vi "poly_lock_fp_updates_unlock_caller.vi"(8 "error in":errorcluster) -> (0 "error out":errorcluster)   [LabVIEW 2015]
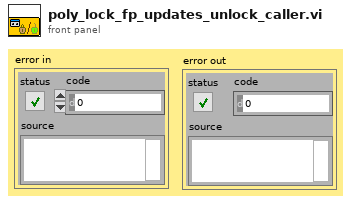
[diagram p1: front panel]
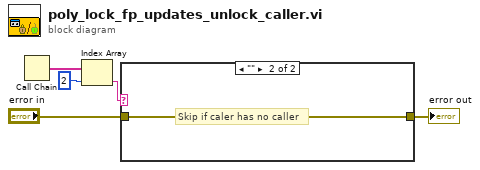
[diagram p0: block diagram]
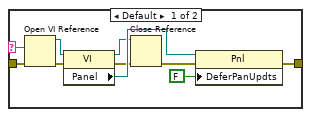
[diagram p2: hidden frame]
diagram:
  n1 = Call Chain() -> (call chain=w3:string[])
  n2 = Index Array(array=w3, index=2) -> (element=w1:string)
  n3 = case shown="\"\"" w1 {
    selector: w1 -> [w12 _]
    tunnel: [w14 w16] -> w5
    tunnel: "error in" -> [w11 w16]
    frame Default {
      n4 = Open VI Reference(vi path=w12, error in (no error)=w11) -> (vi reference=w9:refnum<vi>, error out=w10:errorcluster)  [unwired: 4 in]
      n5 = property class="VI"(reference=w9, error in=w10) -> (reference out=w6:refnum<vi>, error out=w8:errorcluster, "Panel"=w13:refnum<vi>)
      n6 = Close Reference(reference=w6, error in (no error)=w8) -> (error out=w7:errorcluster)
      n7 = property class="Pnl"(reference=w13, error in=w7, "DeferPanUpdts"=FALSE) -> (error out=w14:errorcluster)  [unwired: 1 out]
    }
    frame "" {
      # "Skip if caler has no caller"
    }
  }
  "error out" <- w5
